vi "StopMainGUI.vi"(8 "ErrorIn":errorcluster, 10 "MsTimeout(-1)":i32=-1, 11 "ReferenceIn":refnum<class "JSONTextViewer.lvclass">) -> (0 "ErrorOut":errorcluster, 3 "ReferenceOut":refnum<class "JSONTextViewer.lvclass">)   [LabVIEW 2021, in "JSONTextViewer.lvlib" / "JSONTextViewer.lvclass"]
uses:
  JSONTextViewer.lvclass
  JSONTextViewer.lvclass/JSONTextViewer.ctl
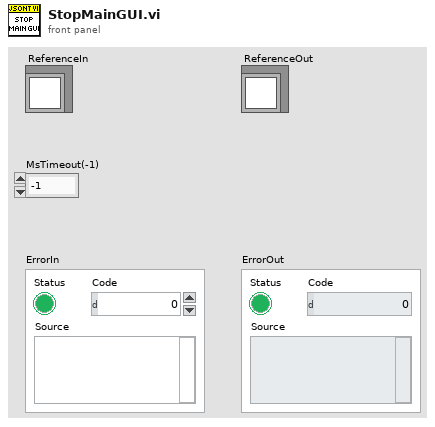
[diagram p1: front panel]
types:
  T1 = enum16{"ReadRepository", "CreateNew", "CreateOrLookUpExisting", "ReadRepositoryAndDestroy"}
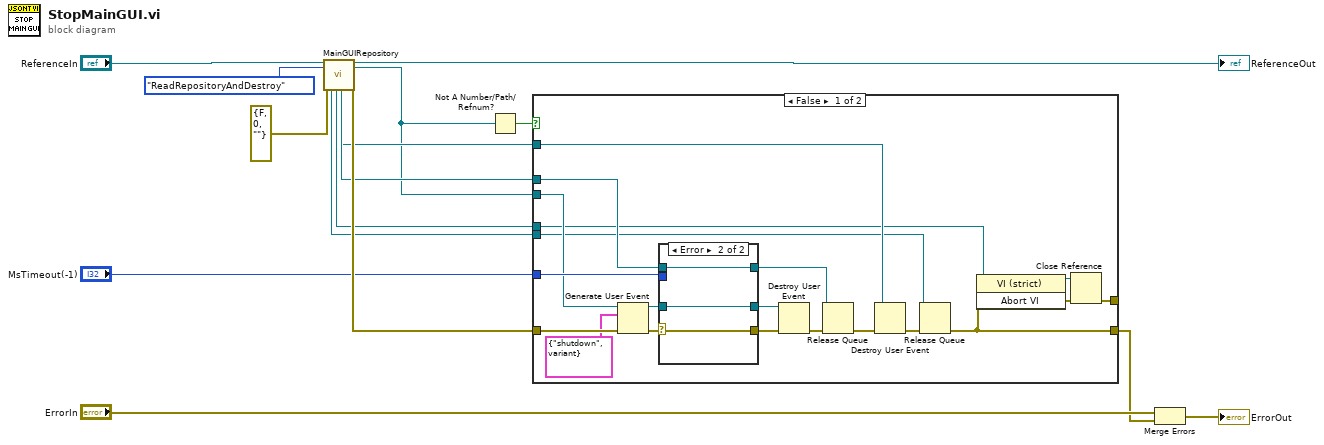
[diagram p0: block diagram]
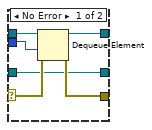
[diagram p2: hidden frame]
diagram:
  n1 = call "MainGUIRepository.vi"("reference in"="ReferenceIn", "Action(ReadRepository)"=T1."ReadRepositoryAndDestroy", "Error In"=errorcluster {"status"=FALSE, "code"=0, "source"=""} ("error in (no error)")) -> ("QueueFromProcess"=w2:refnum<queue>, "ProcessViRef"=w5:refnum<vi>, "EventFromProcess"=w6:refnum<user-event>, "ProcessSyncQueue"=w7:refnum<queue>, "reference out"=→"ReferenceOut":refnum<class "JSONTextViewer.lvclass">, "EventsToProcess"=w4:refnum<user-event>, "Error Out"=w12:errorcluster)  [unwired: 9 in, 1 out]
  n2 = Not A Number/Path/Refnum?(number/path/refnum=w4) -> (NaN/Path/Refnum?=w3:bool)
  n3 = case shown="False" w3 {
    tunnel: w7 -> [w26 _]
    tunnel: w12 -> [w33 w45]
    tunnel: [w27 w45] -> w14
    tunnel: w4 -> [w21 _]
    tunnel: "MsTimeout(-1)" -> [w23 _]
    tunnel: w6 -> [w22 _]
    tunnel: w5 -> [w19 _]
    tunnel: w2 -> [w17 _]
    tunnel: [w28 _] -> _
    frame False {
      n4 = Generate User Event(user event=w21, event data cluster=cluster{"Command":string, "Data":variant} {"Command"="shutdown", "Data"=variant} ("event data"), error in=w33) -> (user event out=w25:refnum<user-event>, error out=w34:errorcluster)  [unwired: 1 in]
      n5 = case shown="Error" w34 {
        tunnel: [w40 w44] -> w35
        tunnel: w26 -> [w38 w42]
        tunnel: [w39 w43] -> w24
        tunnel: w25 -> [w39 w43]
        tunnel: w23 -> [w37 _]
        selector: w34 -> [w41 w44]
        tunnel: [w36 w42] -> w16
        frame No Error {
          n6 = Dequeue Element(queue=w38, timeout in ms (-1)=w37, error in (no error)=w41) -> (queue out=w36:refnum<queue>, error out=w40:errorcluster)  [unwired: 2 out]
        }
        frame Error {
        }
      }
      n7 = Destroy User Event(user event=w24, error in=w35) -> (error out=w30:errorcluster)
      n8 = Release Queue(queue=w16, error in (no error)=w30) -> (error out=w29:errorcluster)  [unwired: 1 in, 2 out]
      n9 = Destroy User Event(user event=w22, error in=w29) -> (error out=w31:errorcluster)
      n10 = Release Queue(queue=w17, error in (no error)=w31) -> (error out=w27:errorcluster)  [unwired: 1 in, 2 out]
      n11 = invoke class="VI (strict)" method="Abort VI"(reference=w19, error in=w27) -> (reference out=w18:refnum<vi>, error out=w32:errorcluster)  [unwired: 1 in, 1 out]
      n12 = Close Reference(reference=w18, error in (no error)=w32) -> (error out=w28:errorcluster)
    }
    frame True {
    }
  }
  n13 = Merge Errors("ErrorIn", w14) -> (→"ErrorOut":errorcluster)
